vi "xxxArray-to-Real-v2.vi"(11 "Numeric in":u32) -> (3 "Numeric out":dbl)   [LabVIEW 2019]
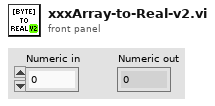
[diagram p1: front panel]
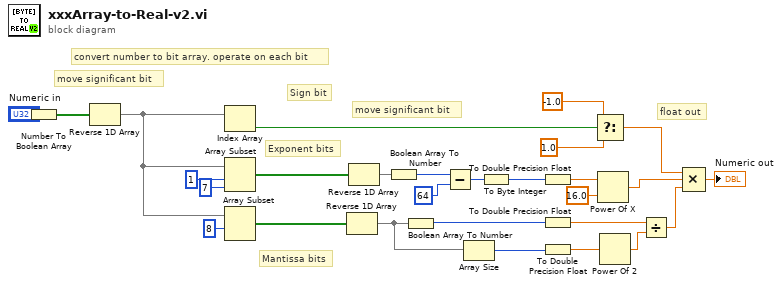
[diagram p0: block diagram]
diagram:
  # "float out"
  # "move significant bit"
  # "Mantissa bits"
  # "move significant bit"
  # "convert number to bit array. operate on each bit"
  # "Exponent bits"
  # "Sign bit"
  n1 = Number To Boolean Array(number="Numeric in") -> (Boolean array=w21:bool[])
  n2 = Reverse 1D Array(array=w21) -> (reversed array=w22:bool[])
  n3 = Index Array(array=w22) -> (element=w6:bool)  [unwired: 1 in]
  n4 = Array Subset(array=w22, index=1, length=7) -> (w23:bool[])
  n5 = Array Subset(array=w22, index=8) -> (w5:bool[])  [unwired: 1 in]
  n6 = Reverse 1D Array(array=w5) -> (reversed array=w26:bool[])
  n7 = Reverse 1D Array(array=w23) -> (reversed array=w18:bool[])
  n8 = Boolean Array To Number(Boolean array=w18) -> (number=w12:u64)
  n9 = Boolean Array To Number(Boolean array=w26) -> (number=w9:u64)
  n10 = Subtract(x=w12, y=u64 64) -> (x-y=w13:u64)
  n11 = Array Size(array=w26) -> (size(s)=w27:i32)
  n12 = To Byte Integer(number=w13) -> (8bit integer=w1:i8)
  n13 = To Double Precision Float(number=w1) -> (double precision float=w25:dbl)
  n14 = To Double Precision Float(number=w9) -> (double precision float=w24:dbl)
  n15 = To Double Precision Float(number=w27) -> (double precision float=w28:dbl)
  n16 = Select(t=-1.0 ("x"), s=w6, f=1.0 ("x")) -> (s? t:f=w15:dbl)
  n17 = Power Of X(1:16.0 ("x"), 2:w25) -> (0:w20:dbl)
  n18 = Power Of 2(x=w28) -> (2^x=w10:dbl)
  n19 = Divide(x=w24, y=w10) -> (x/y=w16:dbl)
  n20 = Compound Arithmetic op=MULTIPLY(w15, w20, w16) -> (→"Numeric out":dbl)
